vi "Scan Engine Custom FPGA Page - ECAT.vi"(8 "error in (no error)":errorcluster, 11 "Node Ptr":T1 format="%.0x") -> (0 "error out":errorcluster)   [LabVIEW 2019, in "SEECD System Explorer.lvlib"]
uses:
  SEECD System Explorer.lvlib
  <vilib>/NI VeriStand/Custom Device API/Custom Device Item Ref.ctl
  Type Defs/FPGA Target.ctl
  <vilib>/NI VeriStand/Custom Device API/Custom Device API.lvlib
panel:
  in  "SHDocVw.IWebBrowser2":refnum<k7>(container)
  out "FPGA Bitfile":path caption="Currently Loaded FPGA Personality"
  in  "Header":cluster{"Section Name":string}={"Section Name"="EtherCAT Slave Custom FPGA Personality Settings"}
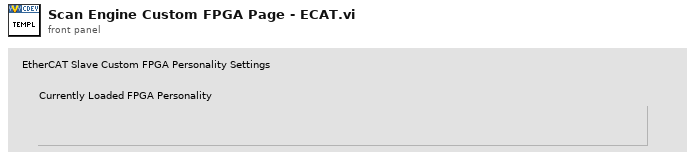
[diagram p1: front panel]
types:
  T1 = typedef "Custom Device API.lvlib/Custom Device Item Ref.ctl" = u64
  T2 = typedef "SEECD System Explorer.lvlib/FPGA Target.ctl" = enum16{"Local", "EtherCAT"}
  T3 = typedef "Custom Device API.lvlib/Custom Device Commands.ctl" = enum16{"Default", "Item renamed", "Shutdown", "Dynamic button pressed"}
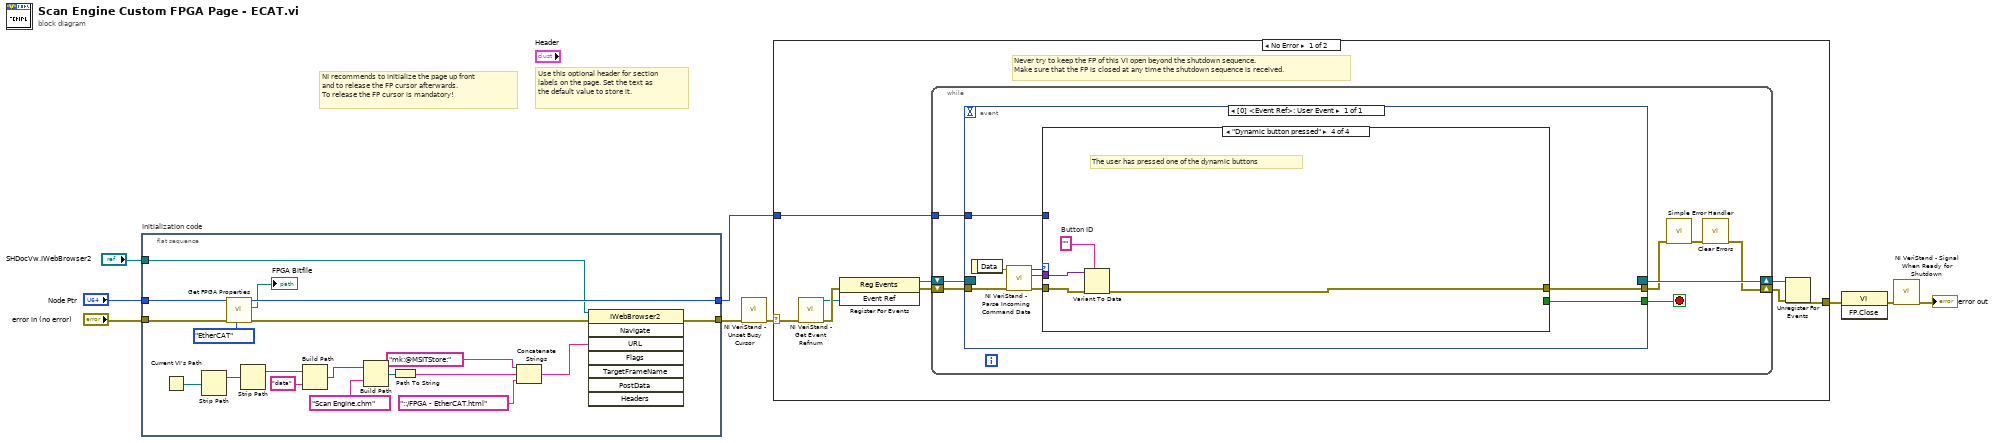
[diagram p0: block diagram]
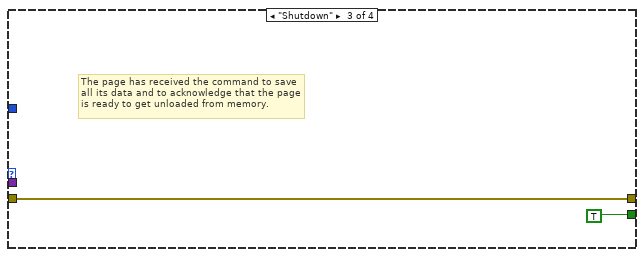
[diagram p4: hidden frame]
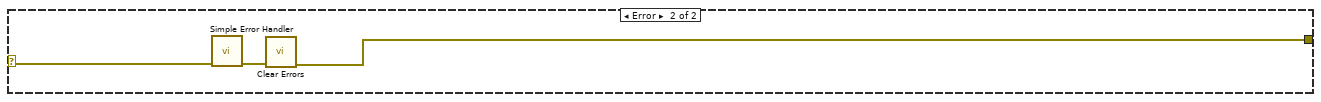
[diagram p5: hidden frame]
diagram:
  # "Use this optional header for section labels on the page. Set the text as the default value to store it."
  # "NI recommends to initialize the page up front\nand to release the FP cursor afterwards.\nTo release the FP cursor is mandatory!"
  n1 = flat-sequence "Initialization code" {
    tunnel: "error in (no error)" -> [w24]
    tunnel: "Node Ptr" -> [w25]
    tunnel: [w13] -> w5
    tunnel: [w28] -> w2
    tunnel: "SHDocVw.IWebBrowser2" -> [w11]
    frame #0 {
      n2 = Current VI's Path() -> (path=w22:path)
      n3 = Strip Path(path=w22) -> (stripped path=w21:path)  [unwired: 1 out]
      n4 = call "Get FPGA Properties.vi"("FPGA Target"=FPGA_Target."EtherCAT", "error in (no error)"=w24, "Item Ref in"=w25) -> ("error out"=w12:errorcluster, "Bitfile Path"=→"FPGA Bitfile":path, "Item Ref out"=w28:T1)  [unwired: 5 in, 1 out]
      n5 = Strip Path(path=w21) -> (stripped path=w16:path)  [unwired: 1 out]
      n6 = Build Path(base path=w16, name or relative path="data") -> (appended path=w15:path)
      n7 = Build Path(base path=w15, name or relative path="Scan Engine.chm") -> (appended path=w18:path)
      n8 = Path To String(path=w18) -> (string=w19:string)
      n9 = Concatenate Strings("mk:@MSITStore:" ("string"), w19, "::/FPGA - EtherCAT.html" ("name or relative path")) -> (w10:string)
      n10 = invoke class="IWebBrowser2" method="Navigate"(reference=w11, error in=w12, "URL"=w10) -> (error out=w13:errorcluster)  [unwired: 5 in, 7 out]
    }
  }
  n11 = call <vilib>:"NI VeriStand - Unset Busy Cursor.vi"("error in (no error)"=w5) -> ("error out"=w4:errorcluster)  [unwired: 10 out]
  n12 = case shown="No Error" w4 {
    selector: w4 -> [w29 w64]
    tunnel: [w34 w62] -> w9
    tunnel: w2 -> [w30 _]
    frame No Error {
      # "Never try to keep the FP of this VI open beyond the shutdown sequence.\nMake sure that the FP is closed at any time the shutdown sequence is received."
      n13 = call <vilib>:"NI VeriStand - Get Event Refnum.vi"("error in (no error)"=w29) -> ("error out"=w37:errorcluster, "Event Ref"=w33:refnum<user-event>)  [unwired: 9 out]
      n14 = register-events(error in=w37, w33) -> (reference out=w31:refnum<event-registration>, error out=w32:errorcluster)  [unwired: 1 in]
      n15 = while {
        tunnel: w30 -> [w41]
        shift-right: [w38] -> w35
        shift-left: w32 -> [w44]
        shift-right: [w45] -> w36
        shift-left: w31 -> [w43]
        stop <- w42 stop-if-true
        n16 = event shown="[0] <Event Ref>: User Event" {
          selector: w43 -> [_]
          dyn-events: [_] -> w45
          timeout: _ -> [_]
          tunnel: w44 -> [w53]
          tunnel: [w49] -> w42
          tunnel: [w48] -> w40
          tunnel: w41 -> [w47]
          event User Event {
            n17 = event-data() -> ("Data"=w52:string)  [unwired: 1 out]
            n18 = call <vilib>:"NI VeriStand - Parse Incoming Command Data.vi"("error in (no error)"=w53, "Incoming data"=w52) -> ("error out"=w51:errorcluster, "Outgoing data"=w46:variant, "Action"=w50:T3)  [unwired: 7 out]
            n19 = case shown="\"Dynamic button pressed\"" w50 {
              tunnel: w51 -> [w54 w55 w56 w61]
              tunnel: [_ _ TRUE _] -> w49
              tunnel: [w54 w55 w56 w58] -> w48
              tunnel: w47 -> [_ _ _ _]
              tunnel: w46 -> [_ _ _ w60]
              frame "Default", Default {
              }
              frame "Item renamed" {
              }
              frame "Shutdown" {
                # "The page has received the command to save all its data and to acknowledge that the page is ready to get unloaded from memory."
              }
              frame "Dynamic button pressed" {
                w59 = ""  # Button ID
                # "The user has pressed one of the dynamic buttons"
                n20 = Variant To Data(error in=w61, type=w59, Variant=w60) -> (error out=w58:errorcluster)  [unwired: 1 out]
              }
            }
          }
        }
        n21 = call <vilib>:"Simple Error Handler.vi"("error in (no error)"=w40) -> ("error out"=w39:errorcluster)  [unwired: 1 in, 7 out]
        n22 = call <vilib>:"Clear Errors.vi"("error in (no error)"=w39) -> ("error out"=w38:errorcluster)  [unwired: 1 in, 5 out]
      }
      n23 = Unregister For Events(event registration refnum=w36, error in=w35) -> (error out=w34:errorcluster)
    }
    frame Error {
      n24 = call <vilib>:"Simple Error Handler.vi"("error in (no error)"=w64) -> ("error out"=w63:errorcluster)  [unwired: 1 in, 7 out]
      n25 = call <vilib>:"Clear Errors.vi"("error in (no error)"=w63) -> ("error out"=w62:errorcluster)  [unwired: 1 in, 5 out]
    }
  }
  n26 = invoke class="VI" method="FP.Close"(error in=w9) -> (error out=w8:errorcluster)  [unwired: 2 in, 2 out]
  n27 = call <vilib>:"NI VeriStand - Signal When Ready for Shutdown.vi"("error in (no error)"=w8) -> ("error out"=→"error out":errorcluster)  [unwired: 10 out]
